vi "SetFreqAndRead.vi"() -> ()   [LabVIEW 2010]
panel:
  out "QY":string
  out "QX":string
  in  "Frequenz":dbl
  in  "error in":errorcluster
  out "error out":errorcluster
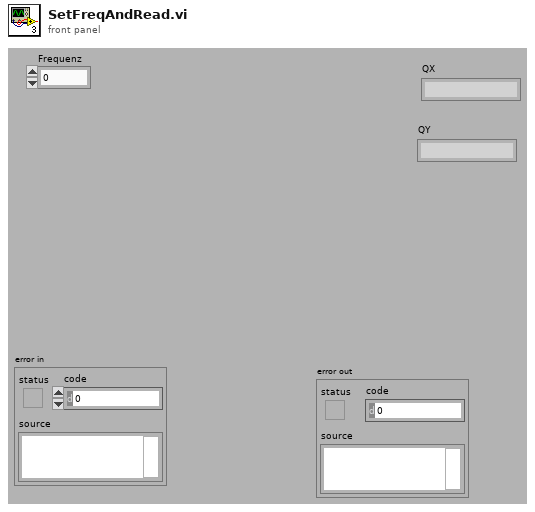
[diagram p1: front panel]
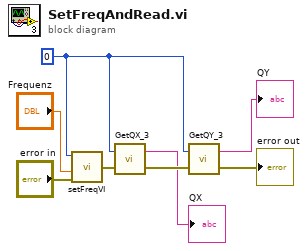
[diagram p0: block diagram]
diagram:
  w1 = 0
  n1 = call "setFreqVI.vi"("error in"="error in", "Frequenz in Hz"="Frequenz", "mode (0)"=w1) -> ("error out"=w8:errorcluster)  [unwired: 1 in]
  n2 = call "GetQX_3.vi"("error in"=w8, "mode (0)"=w1) -> ("error out"=w7:errorcluster, "data"=→"QX":string)
  n3 = call "GetQY_3.vi"("error in"=w7, "mode (0)"=w1) -> ("error out"=→"error out":errorcluster, "data"=→"QY":string)
